vi "Open PDFStamper.vi"(0 "PDF Path (original)":path, 5 "PDF Path (modified )":path, 7 "RotateContents (F)":bool, 9 "Permissions":T2={"User Password"="", "Owner Password"="", "Printing"=enum."Allow Printing", "Allow Modify Contents"=TRUE, "Allow Copy"=TRUE, "Allow Modify Annotations"=TRUE, "Allow Fill In "=TRUE, "Allow Screen Readers"=TRUE, "Allow Assembly"=TRUE}, 11 "error in (no error)":errorcluster, 12 "At the opening":T1={"Page"=1, "Show Bookmarks"=TRUE} {"Page" items=["Single Page - Fit Page"=1, "Single Page - Fit Width"=0]}, 13 "Viewer Preference":i16=-1) -> (4 "PDFStamper":refnum<k24>, 8 "Temporary File Name":path, 10 "NumberOfPages":i32, 15 "error out":errorcluster)   [LabVIEW 2019]
doc: "Version 2.0\nDeveloped by Jean-Marc Simard\nCopyright © 2013, Exaprom Inc.\nAll rights reserved.\nLicense: BSD\n\nWith iTextSharp 4.1.6 (http://itextsharp.sourceforge.net)\nunder Mozilla Public License Version 1.1\n(http://www.mozilla.org/MPL/MPL-1.1.html)"
uses:
  C:/Program Files/National Instruments/LabVIEW 2019/user.lib/Exaprom PDF/DLL/itextsharp.dll
  DLL/itextsharp.dll
  <userlib>/Exaprom PDF/Controls/Initialization Controls/File Permission Parameters.ctl
  <userlib>/Exaprom PDF/Controls/Initialization Controls/At the opening.ctl
  <userlib>/Exaprom PDF/Controls/File Path Controls/Temporary File.ctl
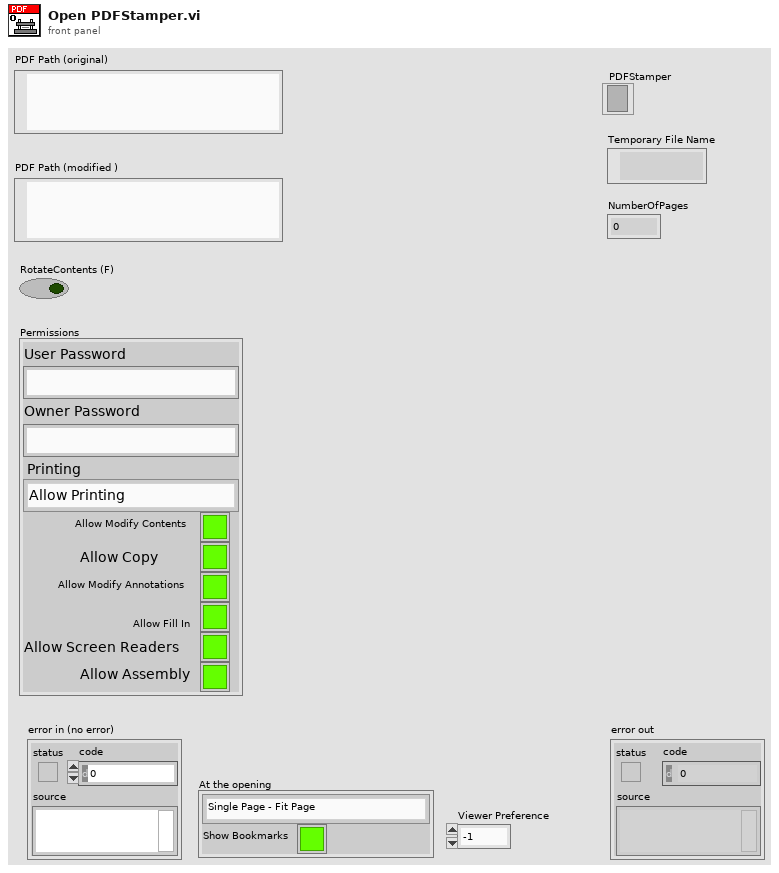
[diagram p1: front panel]
types:
  T1 = typedef "At the opening.ctl" = cluster{"Page":u16, "Show Bookmarks":bool}
  T2 = typedef "File Permission Parameters.ctl" = cluster{"User Password":string, "Owner Password":string, "Printing":enum16{"Allow Printing", "Allow Degraded Printing", "Don't Allow Printing"}, "Allow Modify Contents":bool, "Allow Copy":bool, "Allow Modify Annotations":bool, "Allow Fill In ":bool, "Allow Screen Readers":bool, "Allow Assembly":bool}
  T3 = typedef "Temporary File.ctl" = enum16{".bmp", ".jpeg", ".png", ".pdf", "No File", ".xml"}
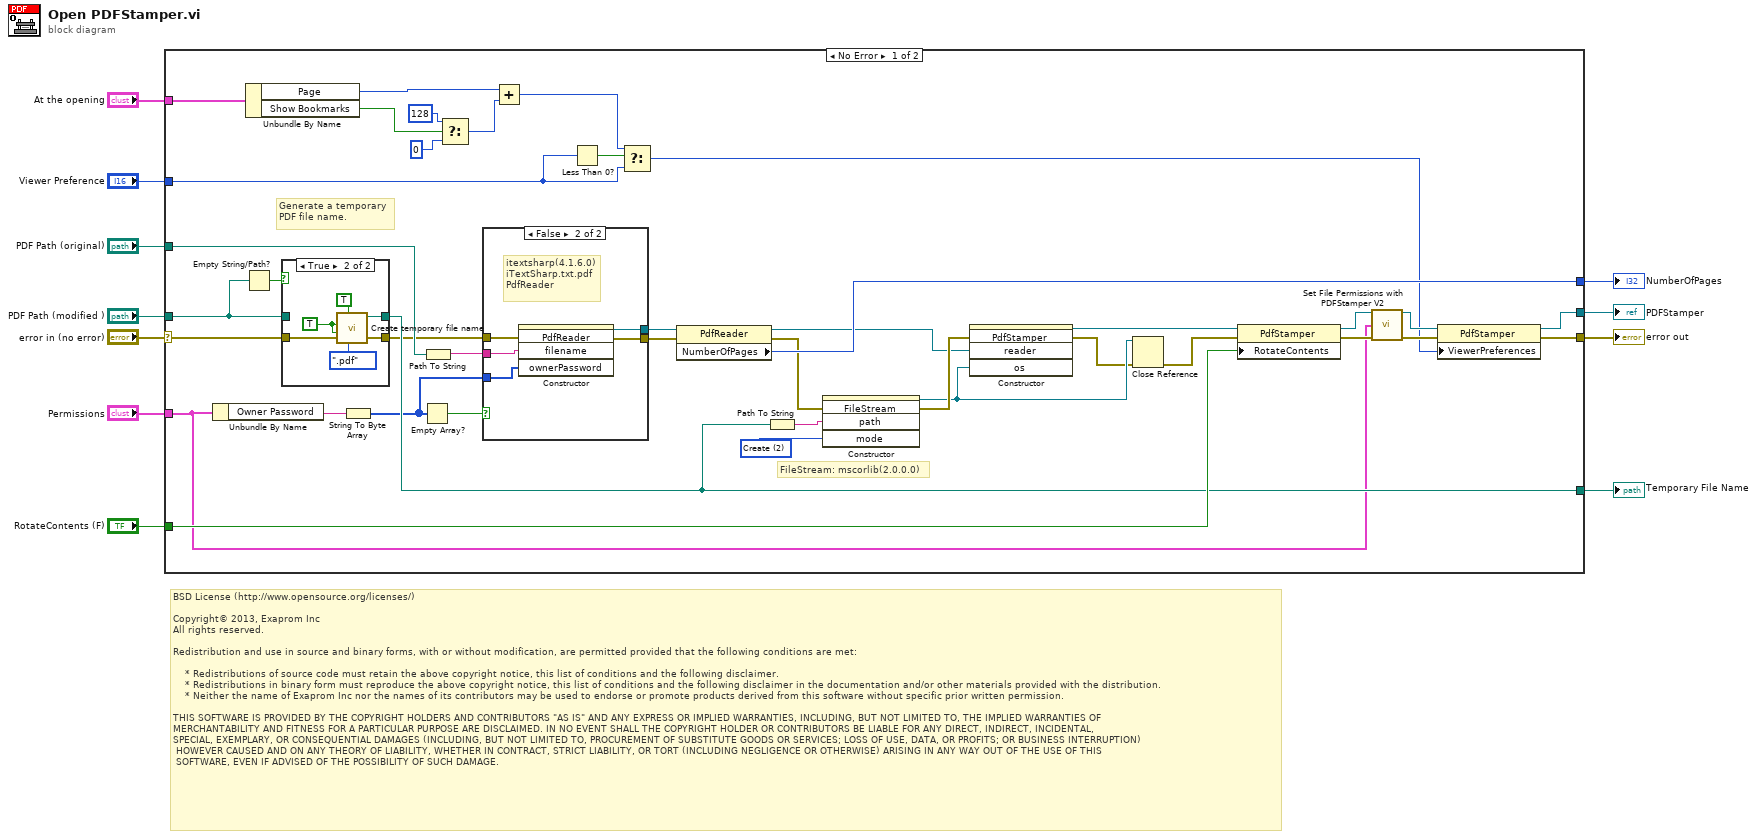
[diagram p0: block diagram]
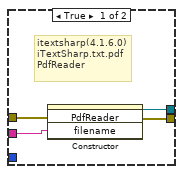
[diagram p3: hidden frame]
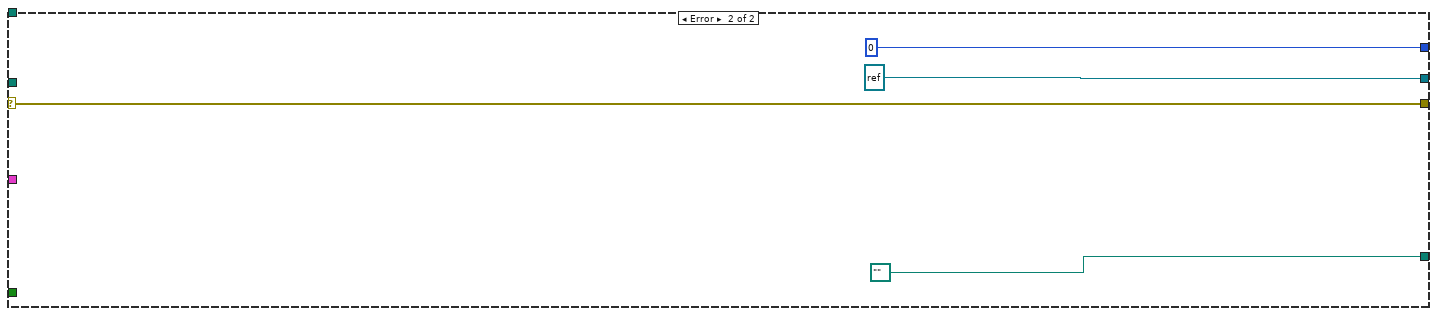
[diagram p4: hidden frame]
diagram:
  # "BSD License (http://www.opensource.org/licenses/)\n\nCopyright© 2013, Exaprom Inc\nAll rights reserved.\n\nRedistribution and use in source and binary forms, with or without modification, are permitted provided that the following conditions are met:\n\n    * Redistributions of source code must retain the above copyright notice, this list of conditions and the following disclaimer.\n    * Redistributions in binary form must reproduce the above copyright notice, this list of conditions and the following disclaimer in the documentation and/or other materials provided with the distribution.\n    * Neither the name of Exaprom Inc nor the names of its contributors may be used to endorse or promote products derived from this software without specific prior written permission.\n\nTHIS SOFTWARE IS PROVIDED BY THE COPYRIGHT HOLDERS AND CONTRIBUTORS \"AS IS\" AND ANY EXPRESS OR IMPLIED WARRANTIES, INCLUDING, BUT NOT LIMITED TO, THE IMPLIED WARRANTIES OF \nMERCHANTABILITY AND FITNESS FOR A PARTICULAR PURPOSE ARE DISCLAIMED. IN NO EVENT SHALL THE COPYRIGHT HOLDER OR CONTRIBUTORS BE LIABLE FOR ANY DIRECT, INDIRECT, INCIDENTAL,\nSPECIAL, EXEMPLARY, OR CONSEQUENTIAL DAMAGES (INCLUDING, BUT NOT LIMITED TO, PROCUREMENT OF SUBSTITUTE GOODS OR SERVICES; LOSS OF USE, DATA, OR PROFITS; OR BUSINESS INTERRUPTION)\n HOWEVER CAUSED AND ON ANY THEORY OF LIABILITY, WHETHER IN CONTRACT, STRICT LIABILITY, OR TORT (INCLUDING NEGLIGENCE OR OTHERWISE) ARISING IN ANY WAY OUT OF THE USE OF THIS\n SOFTWARE, EVEN IF ADVISED OF THE POSSIBILITY OF SUCH DAMAGE."
  n1 = case shown="No Error" "error in (no error)" {
    selector: "error in (no error)" -> [w49 w72]
    tunnel: [w26 w72] -> w9
    tunnel: "PDF Path (original)" -> [w50 _]
    tunnel: [w24 refnum<k24> refnum ("new reference")] -> w7
    tunnel: [w47 0 ("NumberOfPages")] -> w8
    tunnel: "RotateContents (F)" -> [w51 _]
    tunnel: [w48 path "" ("File path")] -> w5
    tunnel: "Permissions" -> [w29 _]
    tunnel: "Viewer Preference" -> [w13 _]
    tunnel: "PDF Path (modified )" -> [w22 _]
    tunnel: "At the opening" -> [w16 _]
    frame No Error {
      w44 = 2 items=["CreateNew"=1, "Create"=2, "Open"=3, "OpenOrCreate"=4, "Truncate"=5, "Append"=6] ("mode")
      # "Generate a temporary\nPDF file name."
      # "FileStream: mscorlib(2.0.0.0)"
      n2 = Unbundle By Name(w29) -> ("Owner Password"=w31:string)
      n3 = Empty String/Path?(string/path=w22) -> (empty?=w23:bool)
      n4 = Unbundle By Name(w16) -> ("Page"=w19:u16, "Show Bookmarks"=w17:bool)
      n5 = case shown="True" w23 {
        tunnel: w49 -> [w52 w59]
        tunnel: [w53 w58] -> w48
        tunnel: [w52 w54] -> w37
        tunnel: w22 -> [w53 _]
        frame False {
        }
        frame True {
          w56 = TRUE ("hh:mm:ss (false)")
          n6 = call <userlib>:"Create temporary file name.vi"("Temporary Image File"=Temporary_File.".pdf", "Flush Files (F)"=TRUE, "error in (no error)"=w59, "msec (F)"=w56, "hh:mm:ss (false)"=w56) -> ("error out"=w54:errorcluster, "File path"=w58:path)  [unwired: 1 in, 4 out]
        }
      }
      n7 = String To Byte Array(string=w31) -> (unsigned byte array=w30:u8[])
      n8 = Empty Array?(array=w30) -> (empty?=w35:bool)
      n9 = Path To String(path=w50) -> (string=w38:string)
      n10 = Select(t=128 ("ViewerPreferences"), s=w17, f=0) -> (s? t:f=w20:i32)
      n11 = case shown="False" w35 {
        tunnel: w38 -> [w63 w68]
        tunnel: w37 -> [w62 w67]
        tunnel: [w61 w66] -> w39
        tunnel: [w60 w65] -> w36
        tunnel: w30 -> [_ w64]
        frame True {
          # "itextsharp(4.1.6.0)\niTextSharp.txt.pdf\nPdfReader"
          n12 = constructor class="PdfReader"(error in=w62, "filename"=w63) -> (reference out=w60:refnum<k24>, error out=w61:errorcluster)  [unwired: 2 in, 2 out]
        }
        frame False {
          # "itextsharp(4.1.6.0)\niTextSharp.txt.pdf\nPdfReader"
          n13 = constructor class="PdfReader"(error in=w67, "filename"=w68, "ownerPassword"=w64) -> (reference out=w65:refnum<k24>, error out=w66:errorcluster)  [unwired: 2 in, 3 out]
        }
      }
      n14 = Add(x=w19, y=w20) -> (x+y=w14:i32)
      n15 = Less Than 0?(x=w13) -> (x < 0?=w15:bool)
      n16 = Select(t=w14, s=w15, f=w13) -> (s? t:f=w12:i32)
      n17 = property class="PdfReader"(reference=w36, error in=w39) -> (reference out=w28:refnum<k24>, error out=w43:errorcluster, "NumberOfPages"=w47:i32)
      n18 = Path To String(path=w48) -> (string=w45:string)
      n19 = constructor class="FileStream"(error in=w43, "path"=w45, "mode"=w44) -> (reference out=w41:refnum<k24>, error out=w46:errorcluster)  [unwired: 2 in, 3 out]
      n20 = constructor class="PdfStamper"(error in=w46, "reader"=w28, "os"=w41) -> (reference out=w27:refnum<k24>, error out=w40:errorcluster)  [unwired: 2 in, 3 out]
      n21 = Close Reference(reference=w41, error in (no error)=w40) -> (error out=w42:errorcluster)
      n22 = property class="PdfStamper"(reference=w27, error in=w42, "RotateContents"=w51) -> (reference out=w34:refnum<k24>, error out=w33:errorcluster)
      n23 = call <userlib>:"Set File Permissions with PDFStamper V2.vi"("PDFStamper IN"=w34, "Permissions"=w29, "error in (no error)"=w33) -> ("PDFStamper OUT"=w25:refnum<k24>, "error out"=w32:errorcluster)  [unwired: 11 in]
      n24 = property class="PdfStamper"(reference=w25, error in=w32, "ViewerPreferences"=w12) -> (reference out=w24:refnum<k24>, error out=w26:errorcluster)
    }
    frame Error {
    }
  }
  "error out" <- w9
  "NumberOfPages" <- w8
  "PDFStamper" <- w7
  "Temporary File Name" <- w5
